vi "Database.vi"(8 "error in (no error)":errorcluster) -> (0 "error out":errorcluster)   [LabVIEW 2017]
uses:
  Type Definitions/Queue FG Options.ctl
  Type Definitions/DB Record.ctl
  Type Definitions/DB Data.ctl
  Type Definitions/DB Info.ctl
  Type Definitions/Controller Message.ctl
  Type Definitions/Controller States.ctl
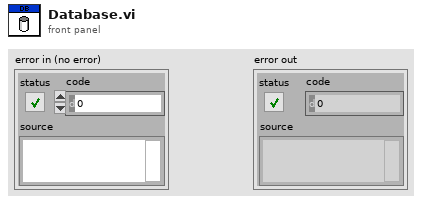
[diagram p1: front panel]
types:
  T1 = typedef "Queue FG Options.ctl" = enum16{"Set", "Get", "Read", "Write", "Destroy"}
  T2 = typedef "DB Data.ctl" = cluster{"Account":i32, "First Name":string, "Last Name":string, "Balance":fxp<+/-,64,35>, "DB Info":T3}
  T3 = typedef "DB Info.ctl" = enum16{"Login Accepted", "Invalid Login", "Deposit Complete", "Withdrawal Complete", "Withdrawal Failed", "Terminate"}
  T4 = typedef "DB Record.ctl" = cluster{"Account":i32, "First Name":string, "Last Name":string, "Balance":fxp<+/-,64,35>}
  T5 = typedef "Controller States.ctl" = enum16{"Initial", "Login", "Idle", "Balance Inquiry", "Deposit", "Withdrawal", "Fast Cash", "Terminate", "Shutdown"}
  T6 = typedef "Controller Message.ctl" = cluster{"Message Info":T5, "Message Data":variant}
  T7 = typedef "Database Message.ctl" = cluster{"Message Info":T8, "Message Data":variant}
  T8 = typedef "Database States.ctl" = enum16{"Initial", "Verify", "Balance Inquiry", "Deposit", "Withdrawal", "Terminate", "Shutdown"}
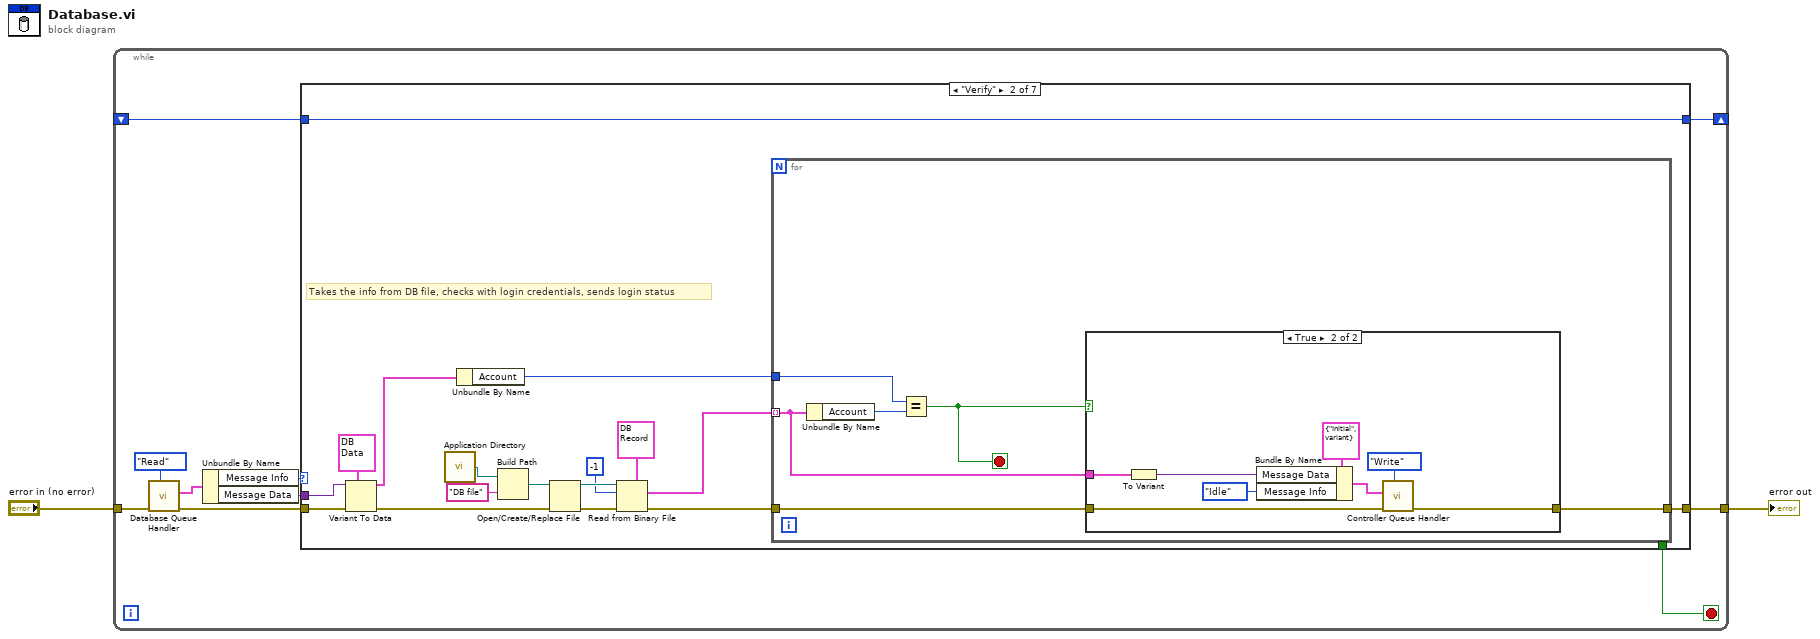
[diagram p0: block diagram]
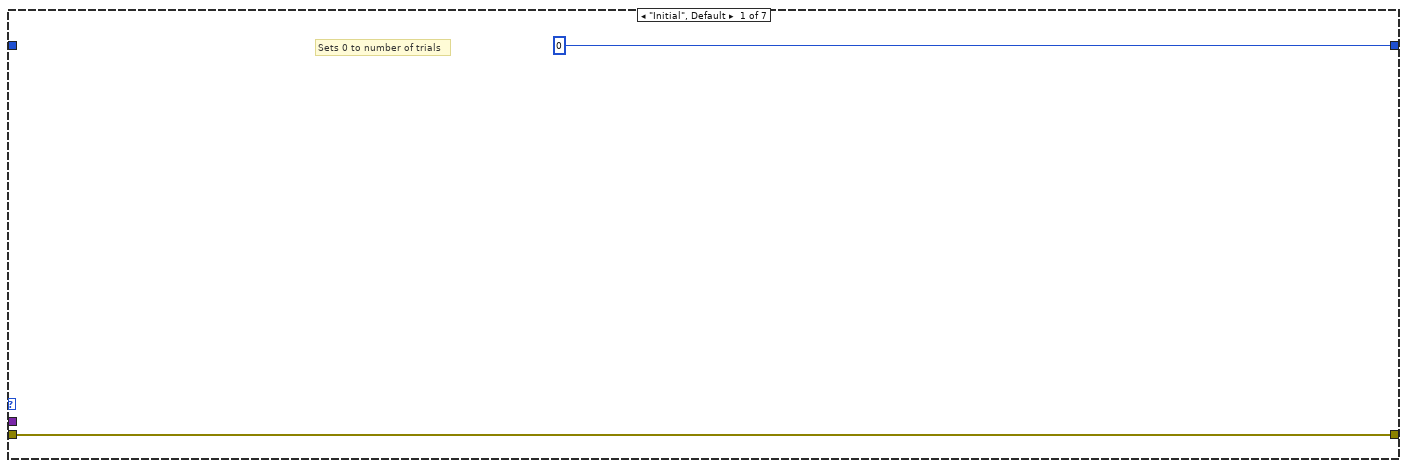
[diagram p2: hidden frame]
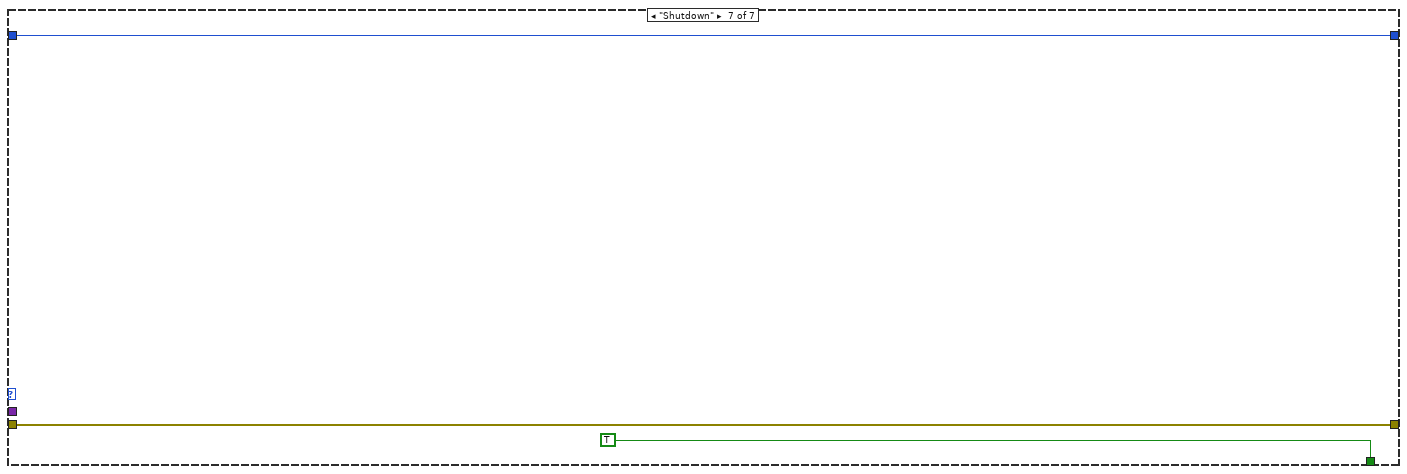
[diagram p8: hidden frame]
diagram:
  n1 = while {
    tunnel: "error in (no error)" -> [w11]
    tunnel: [w6] -> w1
    shift-right: [w4] -> _
    shift-left: _ -> [w3]
    stop <- w5 stop-if-true
    n2 = call "Database Queue Handler.vi"("Action"=Queue_FG_Options."Read", "error in (no error)"=w11) -> ("error out"=w7:errorcluster, "Message out"=w10:T7)  [unwired: 7 in, 1 out]
    n3 = Unbundle By Name(w10) -> ("Message Info"=w9:T8, "Message Data"=w8:variant)
    n4 = case shown="\"Verify\"" w9 {
      tunnel: w8 -> [_ w21 _ _ _ _ _]
      tunnel: w7 -> [w14 w24 w48 w50 w52 w54 w57]
      tunnel: [w14 w15 w48 w50 w52 w54 w57] -> w6
      tunnel: [_ _ _ _ _ _ TRUE] -> w5
      tunnel: [0 w31 w47 w49 w51 w53 w55] -> w4
      tunnel: w3 -> [_ w31 w47 w49 w51 w53 w55]
      frame "Initial", Default {
        # "Sets 0 to number of trials"
      }
      frame "Verify" {
        # "Takes the info from DB file, checks with login credentials, sends login status"
        n5 = Variant To Data(error in=w24, type=T2 {"Account"=0, "First Name"="", "Last Name"="", "Balance"=0.0, "DB Info"=enum."Login Accepted"} ("DB Data in"), Variant=w21) -> (data=w19:T2, error out=w22:errorcluster)
        n6 = call <vilib>:"Application Directory.vi"() -> ("Application Directory"=w30:path)
        n7 = Unbundle By Name(w19) -> ("Account"=w18:i32)
        n8 = Build Path(base path=w30, name or relative path="DB file") -> (appended path=w28:path)
        n9 = Open/Create/Replace File(file path (use dialog)=w28, error in=w22) -> (refnum out=w27:refnum<file>, error out=w23:errorcluster)  [unwired: 4 in, 1 out]
        n10 = Read from Binary File(5:T4 {"Account"=0, "First Name"="", "Last Name"="", "Balance"=0.0} ("DB Record"), 8:w23, 10:-1 ("count (1)"), 11:w27) -> (0:w16:errorcluster, 2:w17:T4[])  [unwired: 2 in, 2 out]
        n11 = for {
          tunnel: w18 -> [w36]
          tunnel: w17 -> [w32] mode=indexing
          tunnel: w16 -> [w35]
          tunnel: [w34] -> w15
          stop <- w33 stop-if-true
          n12 = Unbundle By Name(w32) -> ("Account"=w37:i32)
          n13 = Equal?(x=w36, y=w37) -> (x = y?=w33:bool)
          n14 = case shown="True" w33 {
            tunnel: w35 -> [w38 w46]
            tunnel: [w38 w45] -> w34
            tunnel: w32 -> [_ w40]
            frame False {
            }
            frame True {
              n15 = To Variant(anything=w40) -> (Variant=w39:variant)
              n16 = Bundle By Name(cluster=T6 {"Message Info"=enum."Initial", "Message Data"=variant} ("Message"), "Message Data"=w39, "Message Info"=Controller_States."Idle") -> (w42:T6)
              n17 = call "Controller Queue Handler.vi"("Action"=Queue_FG_Options."Write", "error in (no error)"=w46, "Message in"=w42) -> ("error out"=w45:errorcluster)  [unwired: 6 in, 2 out]
            }
          }
        }
      }
      frame "Balance Inquiry" {
        # "Sends the current account state"
      }
      frame "Deposit" {
        # "Adds amount of money to the account"
      }
      frame "Withdrawal" {
        # "Subtracts amount of money from the account"
      }
      frame "Terminate" {
        # "Sends information Terminate to Controller"
      }
      frame "Shutdown" {
      }
    }
  }
  "error out" <- w1
